vi "Do Read.vi"(8 "error in (no error)":errorcluster, 10 "Interface":refnum<class "Interface.lvclass">, 11 "Section in":refnum<class "Section.lvclass">) -> (0 "error out":errorcluster, 2 "All Keys Found?":bool, 3 "Section out":refnum<class "Section.lvclass">)   [LabVIEW 2015, in "Configuration.lvlib" / "Section.lvclass"]
doc: "Read keys/value pairs from Interface.\n\nProtected dynamic dispatch VI to be overwritten by derived classes."
uses:
  Section.lvclass
  Interface/Interface.lvclass
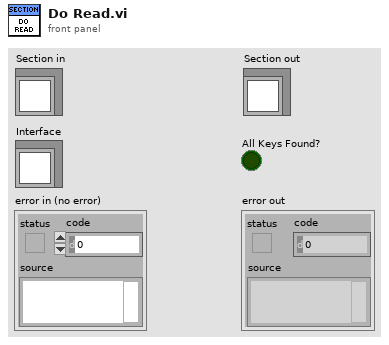
[diagram p1: front panel]
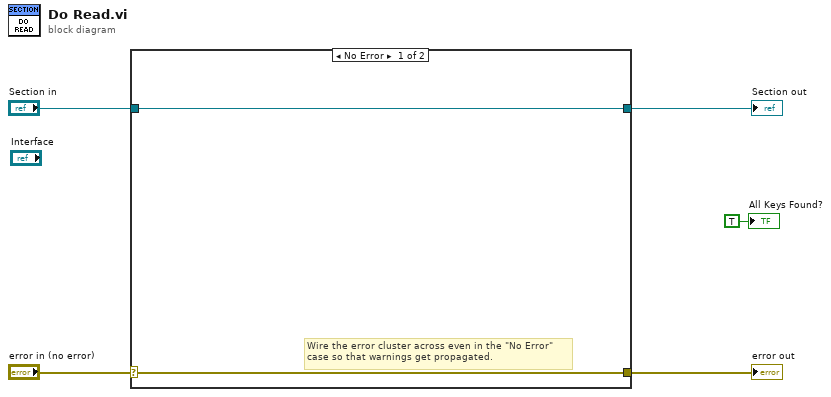
[diagram p0: block diagram]
diagram:
  n1 = case shown="No Error" "error in (no error)" {
    selector: "error in (no error)" -> [w7 w9]
    tunnel: [w7 w9] -> w4
    tunnel: [w6 w8] -> w2
    tunnel: "Section in" -> [w6 w8]
    frame No Error {
      # "Wire the error cluster across even in the \"No Error\"\ncase so that warnings get propagated."
    }
    frame Error {
    }
  }
  "error out" <- w4
  "Section out" <- w2
  "All Keys Found?" <- TRUE ("All Keys Found?")
